vi "Read_PanelBounds.vi"(4 "bot":i32=720, 5 "top":i32=100, 6 "right":i32=1100, 7 "left":i32=200, 10 "path":path, 11 "refnum in":T1) -> (3 "refnum out":T1)   [LabVIEW 2015]
uses:
  <vilib>/Utility/config.llb/Config Data RefNum.ctl
  <vilib>/Utility/config.llb/Read Key (I32).vi
  <vilib>/Utility/config.llb/NI_LVConfig.lvlib
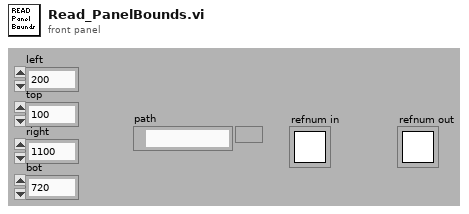
[diagram p1: front panel]
types:
  T1 = typedef "NI_LVConfig.lvlib/Config Data RefNum.ctl" = refnum<k1>
  T2 = cluster{"value":i32, "value":i32, "value":i32, "value":i32}
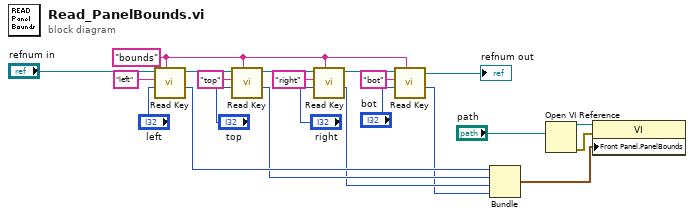
[diagram p0: block diagram]
diagram:
  w20 = "bounds" ("section")
  n1 = call-poly <vilib>:"Read Key.vi"("section"=w20, "default value"="left", "key"="left", "refnum"="refnum in") -> ("value"=w5:i32, "refnum out"=w19:T1)  [unwired: 4 in, 2 out]
  n2 = call-poly <vilib>:"Read Key.vi"("section"=w20, "default value"="top", "key"="top", "refnum"=w19) -> ("value"=w3:i32, "refnum out"=w17:T1)  [unwired: 4 in, 2 out]
  n3 = call-poly <vilib>:"Read Key.vi"("section"=w20, "default value"="right", "key"="right", "refnum"=w17) -> ("value"=w2:i32, "refnum out"=w16:T1)  [unwired: 4 in, 2 out]
  n4 = call-poly <vilib>:"Read Key.vi"("section"=w20, "default value"="bot", "key"="bot", "refnum"=w16) -> ("value"=w1:i32, "refnum out"=→"refnum out":T1)  [unwired: 4 in, 2 out]
  n5 = Bundle("value"=w5, "value"=w3, "value"=w2, "value"=w1) -> (w4:T2)  [unwired: 1 in]
  n6 = Open VI Reference(vi path="path") -> (vi reference=w12:refnum<vi>, error out=w11:errorcluster)  [unwired: 5 in]
  n7 = property class="VI"(reference=w12, error in=w11, "Front Panel.PanelBounds"=w4) -> ()  [unwired: 2 out]
